vi "_023.vi"() -> ()   [LabVIEW 2024]
uses:
  <vilib>/numeric/Random Number (Range) U64.vi
  <vilib>/numeric/sub_Random U32.vi
panel:
  out "Waveform Graph":u64[](graph)
  in  "stop":bool
  out "Waveform Chart":u64(graph)
  # "Chart & Graph"
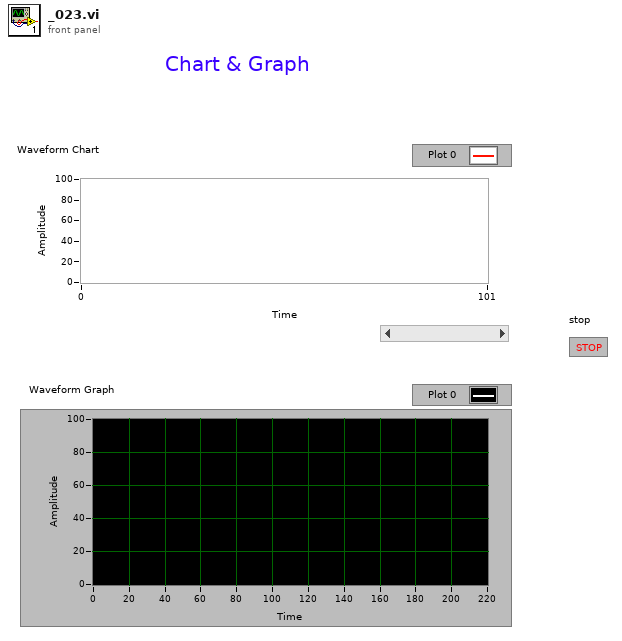
[diagram p1: front panel]
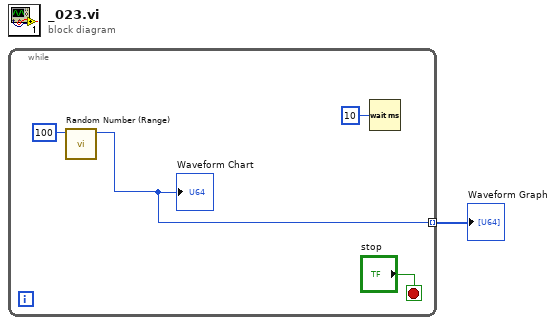
[diagram p0: block diagram]
diagram:
  n1 = while {
    tunnel: [w2] -> w1 mode=indexing
    stop <- "stop" stop-if-true
    n2 = call-poly <vilib>:"Random Number (Range).vi"("upper bound (100)"=u64 100) -> ("number"=w2:u64)  [unwired: 10 in]
    "Waveform Chart" <- w2
    n3 = Wait (ms)(milliseconds to wait=u32 10 ("millisecond timer value")) -> ()  [unwired: 1 out]
  }
  "Waveform Graph" <- w1
